vi "全局2.vi"() -> ()   [LabVIEW 2020]
panel:
  out "右标定":dbl
  out "左标定":dbl
  out "右加载":dbl
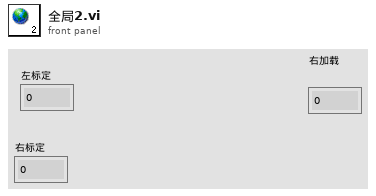
[diagram p1: front panel]
diagram:
